vi "makeTargetPlots.vi"(5 "nPoints":i32, 7 "ZrefMSmm":dbl, 9 "Cluster":T1={"Code"="", "n"=0.0, "Z:FS:(m)"=[], "U:FS:(m/s)"=[15.0, 25.5], "TI::(%)"=[15.0, 25.5]} {"n" min=0.02 max=0.5 step=0.01 format="%.2f"}, 10 "Fit Zmax":dbl, 11 "Fit Zmin":dbl) -> (0 "Code":string, 2 "TIzClusterOut":cluster{"TI::(%)":dbl[], "Array":dbl[]}, 3 "UzClusterOutput":cluster{dbl[], dbl[]})   [LabVIEW 2021]
uses:
  BLTarget.ctl
  Results_plotter_Global.vi
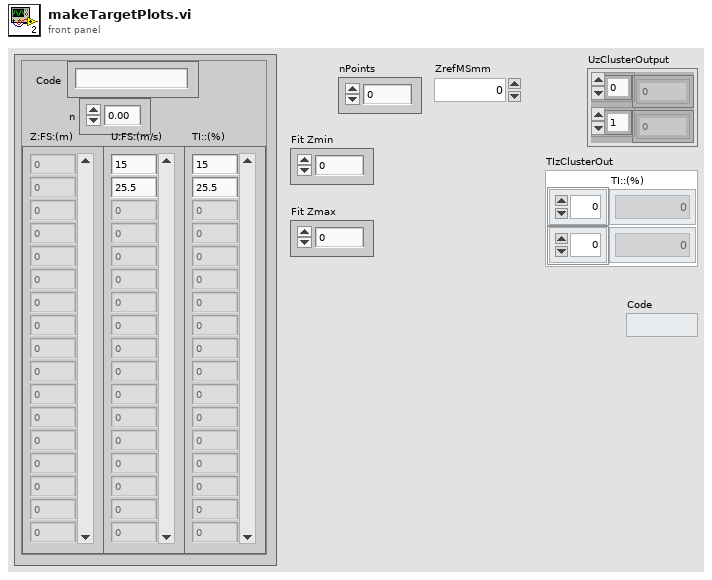
[diagram p1: front panel]
types:
  T1 = typedef "BLTarget.ctl" = cluster{"Code":string, "n":dbl, "Z:FS:(m)":dbl[], "U:FS:(m/s)":dbl[], "TI::(%)":dbl[]}
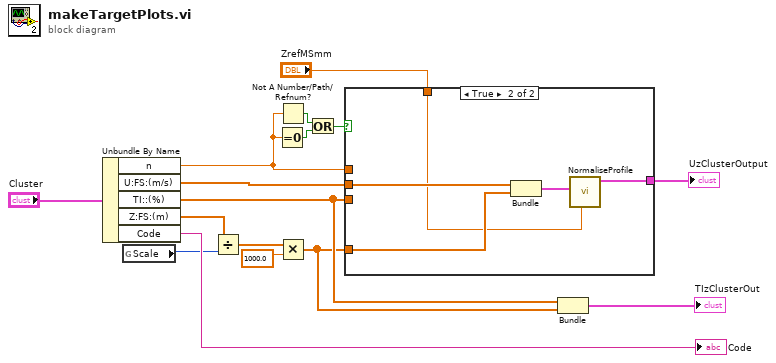
[diagram p0: block diagram]
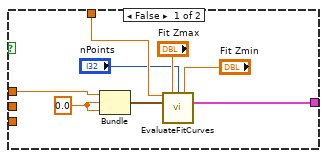
[diagram p2: hidden frame]
diagram:
  n1 = Unbundle By Name("Cluster") -> ("n"=w3:dbl, "U:FS:(m/s)"=w11:dbl[], "TI::(%)"=w7:dbl[], "Z:FS:(m)"=w12:dbl[], "Code"=→"Code":string)
  n2 = global read "Results_plotter_Global.vi" "Scale"() -> (w13:u16)
  n3 = Divide(x=w12, y=w13) -> (x/y=w16:dbl[])
  n4 = Equal To 0?(x=w3) -> (x = 0?=w8:bool)
  n5 = Not A Number/Path/Refnum?(number/path/refnum=w3) -> (NaN/Path/Refnum?=w1:bool)
  n6 = Multiply(x=w16, y=1000.0) -> (x*y=w6:dbl[])
  n7 = Or(x=w1, y=w8) -> (x .or. y?=w2:bool)
  n8 = case shown="True" w2 {
    tunnel: w7 -> [_ _]
    tunnel: w6 -> [_ w29]
    tunnel: w11 -> [_ w28]
    tunnel: [w22 w26] -> w9
    tunnel: "ZrefMSmm" -> [w21 w25]
    tunnel: w3 -> [w23 _]
    frame False {
      w17 = 0.0 ("d0")
      n9 = Bundle("n"=w23, "d0"=w17, "d0"=w17) -> (w20:cluster{"n":dbl, "d0":dbl, "d0":dbl})  [unwired: 1 in]
      n10 = call "EvaluateFitCurves.vi"("Zref"=w21, "Fit Zmax"="Fit Zmax", "nPoints"="nPoints", "Fit Zmin"="Fit Zmin", "PowerLaw"=w20) -> ("PlotCluster"=w22:cluster{"Array":dbl[], "Array":dbl[]})  [unwired: 10 in]
    }
    frame True {
      n11 = Bundle("U:FS:(m/s)"=w28, w29) -> (w27:cluster{"U:FS:(m/s)":dbl[], dbl[]})  [unwired: 1 in]
      n12 = call "NormaliseProfile.vi"("Zref"=w25, "UzClusterIn"=w27) -> ("UzClusterOutput"=w26:cluster{dbl[], dbl[]})  [unwired: 8 in, 1 out]
    }
  }
  "UzClusterOutput" <- w9
  n13 = Bundle("TI::(%)"=w7, w6) -> (→"TIzClusterOut":cluster{"TI::(%)":dbl[], dbl[]})  [unwired: 1 in]
